vi "InitUI.vi"(8 "error in (no error)":errorcluster, 11 "View in":refnum<class "View.lvclass">) -> (0 "error out":errorcluster, 3 "View out":refnum<class "View.lvclass">)   [LabVIEW 2024, in "GUI.lvlib" / "View.lvclass"]
uses:
  View.lvclass
  View.lvclass/View.ctl
  Buttons/ButtonBlack.ctl
  Controller/Controller.lvclass
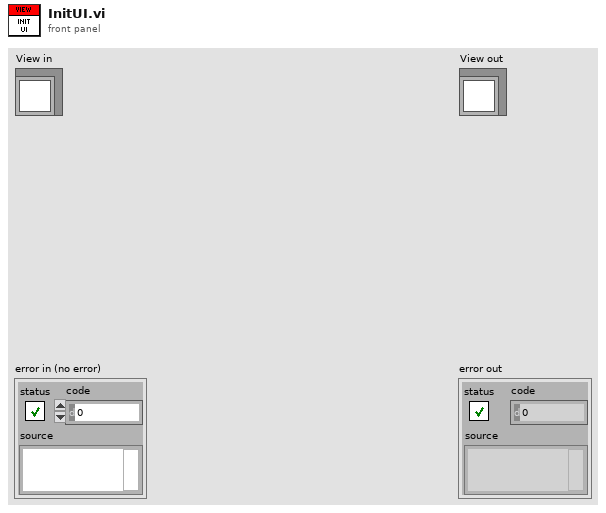
[diagram p1: front panel]
types:
  T1 = typedef "ButtonBlack.ctl" = bool
  T2 = typedef "Settings.ctl" = cluster{"Difficulty":i32}
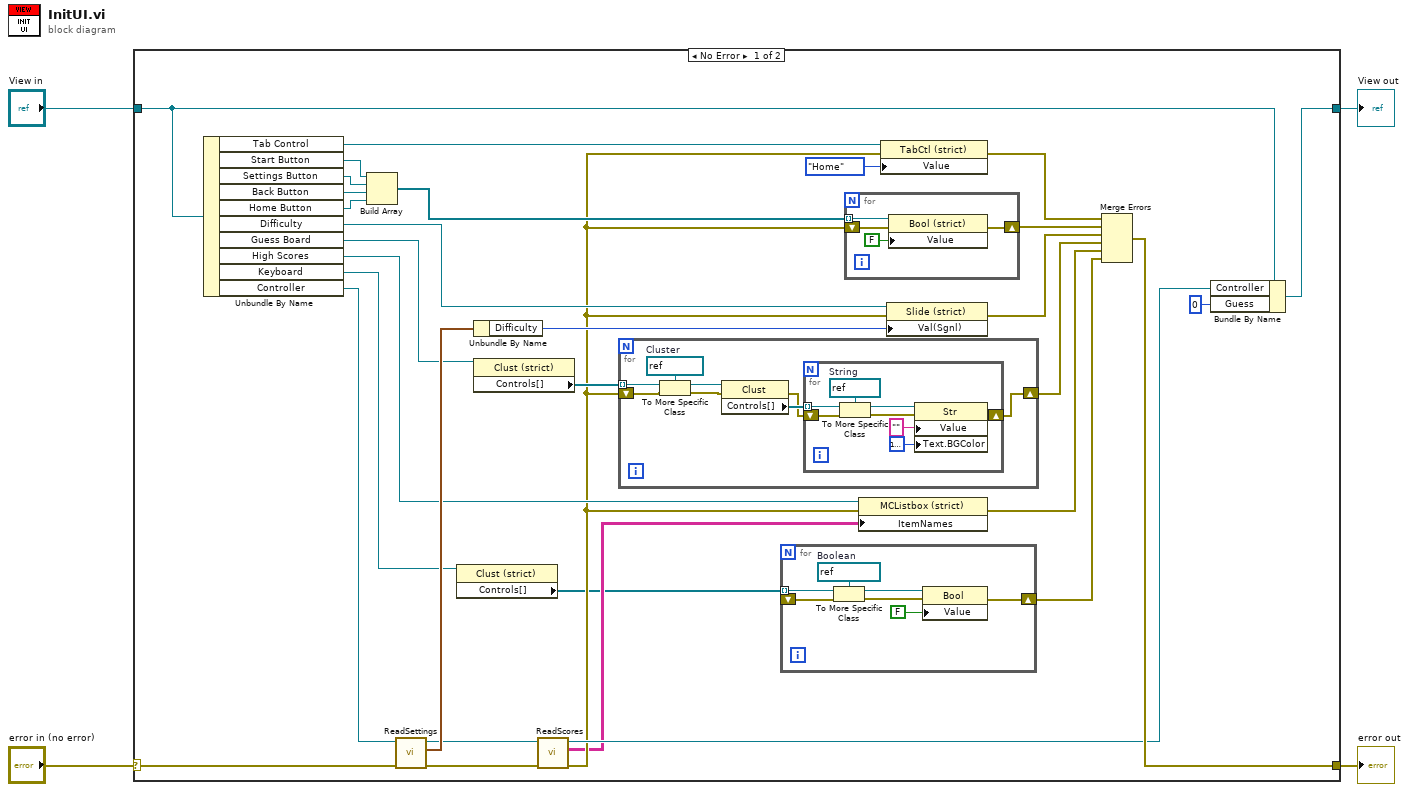
[diagram p0: block diagram]
diagram:
  n1 = case shown="No Error" "error in (no error)" {
    selector: "error in (no error)" -> [w25 w65]
    tunnel: [w27 w65] -> w3
    tunnel: [w19 w64] -> w1
    tunnel: "View in" -> [w20 w64]
    frame No Error {
      n2 = Unbundle By Name(w20) -> ("Tab Control"=w36:refnum<vi>, "Start Button"=w34:refnum<vi>, "Settings Button"=w33:refnum<vi>, "Back Button"=w32:refnum<vi>, "Home Button"=w31:refnum<vi>, "Difficulty"=w24:refnum<vi>, "Guess Board"=w18:refnum<vi>, "High Scores"=w15:refnum<vi>, "Keyboard"=w8:refnum<vi>, "Controller"=w26:refnum<class "Controller.lvclass">)
      n3 = Build Array(w34, w33, w32, w31) -> (w30:refnum<vi>[])
      n4 = call "ReadSettings.vi"("error in (no error)"=w25, "Controller in"=w26) -> ("error out"=w12:errorcluster, "Settings"=w23:T2, "Controller out"=w13:refnum<class "Controller.lvclass">)  [unwired: 7 in]
      n5 = property class="Clust (strict)"(reference=w8) -> ("Controls[]"=w7:refnum<vi>[])  [unwired: 1 in, 2 out]
      n6 = Unbundle By Name(w23) -> ("Difficulty"=w22:i32)
      n7 = property class="Clust (strict)"(reference=w18) -> ("Controls[]"=w17:refnum<vi>[])  [unwired: 1 in, 2 out]
      n8 = call "ReadScores.vi"("error in (no error)"=w12, "Controller in"=w13) -> ("error out"=w10:errorcluster, "Scores"=w9:string[][], "Controller out"=w11:refnum<class "Controller.lvclass">)  [unwired: 7 in]
      n9 = for {
        tunnel: w17 -> [w48] mode=indexing
        shift-right: [w51] -> w16
        shift-left: w10 -> [w49]
        w50 = refnum<vi> refnum  # Cluster
        n10 = To More Specific Class(target class=w50, reference=w48, error in=w49) -> (specific class reference=w47:refnum<vi>, error out=w46:errorcluster)
        n11 = property class="Clust"(reference=w47, error in=w46) -> (error out=w44:errorcluster, "Controls[]"=w45:refnum<vi>[])  [unwired: 1 out]
        n12 = for {
          tunnel: w45 -> [w55] mode=indexing
          shift-right: [w59] -> w51
          shift-left: w44 -> [w54]
          w56 = refnum<vi> refnum  # String
          n13 = To More Specific Class(target class=w56, reference=w55, error in=w54) -> (specific class reference=w52:refnum<vi>, error out=w53:errorcluster)
          n14 = property class="Str"(reference=w52, error in=w53, "Value"="", "Text.BGColor"=u32 16777225 ("Text.Text Colors:BG Color")) -> (error out=w59:errorcluster)  [unwired: 1 out]
        }
      }
      n15 = for {
        tunnel: w7 -> [w41] mode=indexing
        shift-right: [w38] -> w6
        shift-left: _ -> [w42]
        w43 = refnum<vi> refnum  # Boolean
        n16 = To More Specific Class(target class=w43, reference=w41, error in=w42) -> (specific class reference=w40:refnum<vi>, error out=w39:errorcluster)
        n17 = property class="Bool"(reference=w40, error in=w39, "Value"=T1 FALSE) -> (error out=w38:errorcluster)  [unwired: 1 out]
      }
      n18 = for {
        tunnel: w30 -> [w63] mode=indexing
        shift-right: [w61] -> w29
        shift-left: w10 -> [w60]
        n19 = property class="Bool (strict)"(reference=w63, error in=w60, "Value"=T1 FALSE) -> (error out=w61:errorcluster)  [unwired: 1 out]
      }
      n20 = property class="MCListbox (strict)"(reference=w15, error in=w10, "ItemNames"=w9) -> (error out=w14:errorcluster)  [unwired: 1 out]
      n21 = property class="TabCtl (strict)"(reference=w36, error in=w10, "Value"=enum32{"Home", "Settings", "Game", "Scores"}."Home") -> (error out=w28:errorcluster)  [unwired: 1 out]
      n22 = property class="Slide (strict)"(reference=w24, error in=w10, "Val(Sgnl)"=w22) -> (error out=w21:errorcluster)  [unwired: 1 out]
      n23 = Merge Errors(w28, w29, w21, w16, w14, w6) -> (w27:errorcluster)
      n24 = Bundle By Name(cluster=w20, "Controller"=w11, "Guess"=0) -> (w19:refnum<class "View.lvclass">)
    }
    frame Error {
    }
  }
  "error out" <- w3
  "View out" <- w1
